vi "Change Camera.vi"() -> ()   [LabVIEW 2015]
uses:
  <vilib>/Rock Robotics/SystemInterfaces/NetworkCommunication/NetComm_UsageReport_ResourceType.ctl
panel:
  in  "error in (no error)":errorcluster
  in  "Switch Camera 2":bool
  in  "Switch Camera":bool
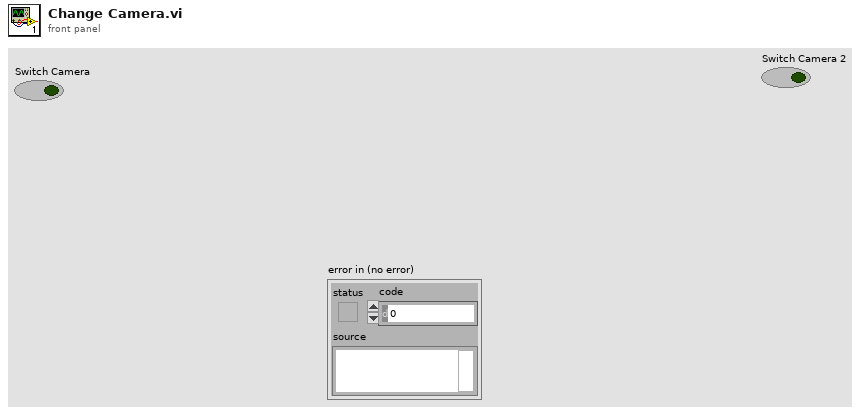
[diagram p1: front panel]
types:
  T1 = cluster{"fps":i32, "compression":i32, "compression 2":i32}
  T2 = typedef "NetComm_UsageReport_ResourceType.ctl" = enum8{"Controller", "Module", "Language", "CANPlugin", "Accelerometer", "ADXL345", "AnalogChannel", "AnalogTrigger", "AnalogTriggerOutput", "CANJaguar", "Compressor", "Counter", "Dashboard", "DigitalInput", "DigitalOutput", "DriverStationCIO", "DriverStationEIO", "DriverStationLCD", "Encoder", "GearTooth", "Gyro", "I2C", "Framework", "Jaguar", "Joystick", "Kinect", "KinectStick", "PIDController", "Preferences", "PWM", "Relay", "RobotDrive", "SerialPort", "Servo", "Solenoid", "SPI", "Task", "Ultrasonic", "Victor", "Button", "Command", "AxisCamera", "PCVideoServer", "SmartDashboard", "Talon", "HiTechnicColorSensor", "HiTechnicAccel", "HiTechnicCompass", "SRF08", "AnalogOutput", "Victor SP", "Talon SRX", "CAN Talon SRX", "ADXL362 Accel", "ADXRS450 Gyro", "Rev SPARK", "Mindsensors SD540", "Digital Filter"}
  T3 = enum16{"Update Mode", "Get Image", "Get Image Data"}
  T4 = typedef "WPI_CameraDevRef.ctl" = cluster{"Camera Address":string, "CameraStatus":errorcluster}
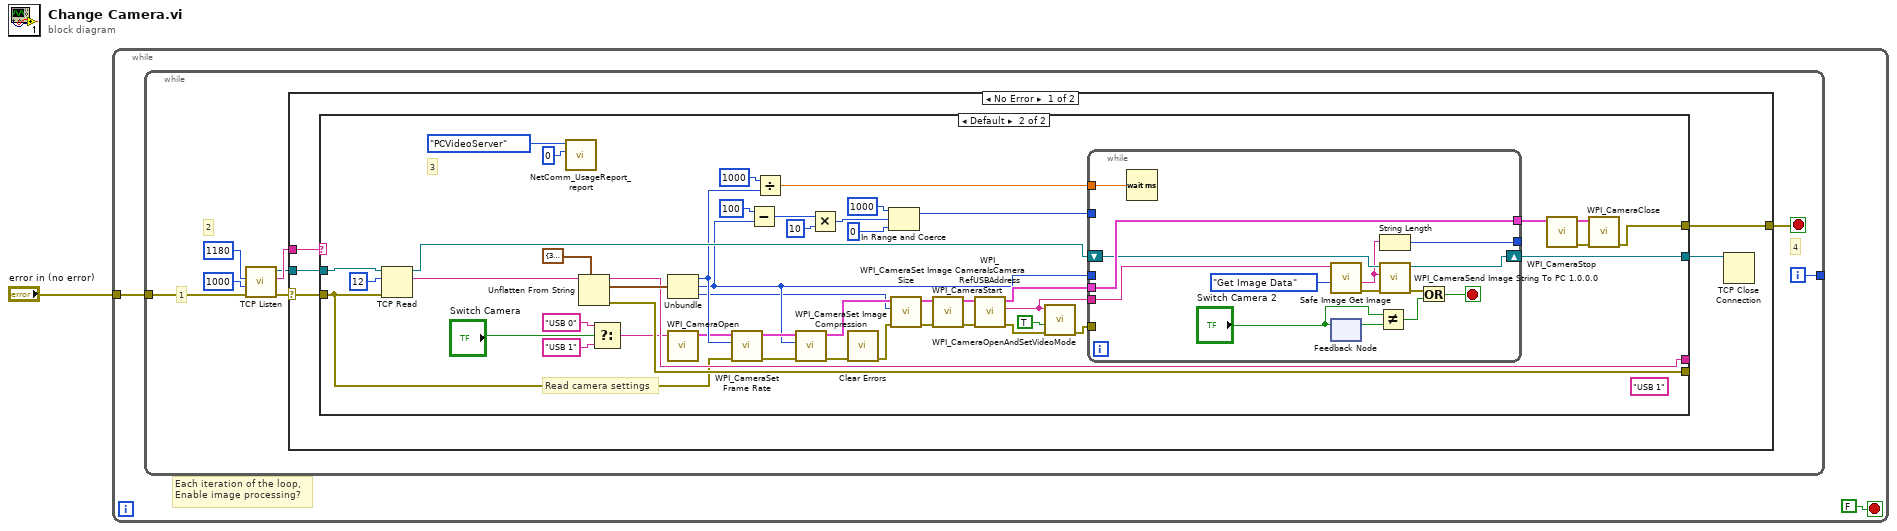
[diagram p0: block diagram]
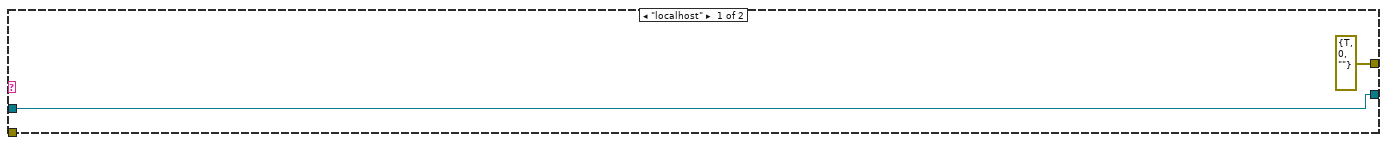
[diagram p2: hidden frame]
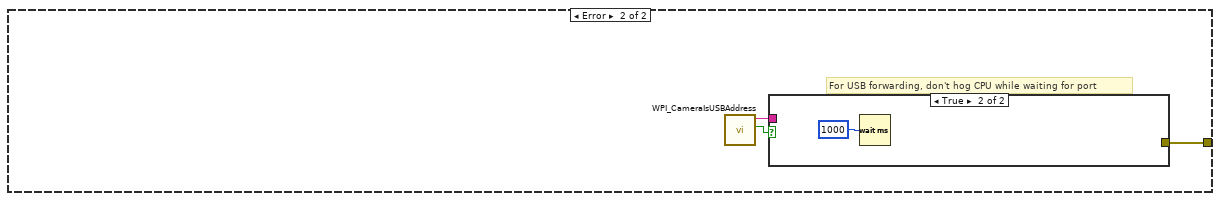
[diagram p3: hidden frame]
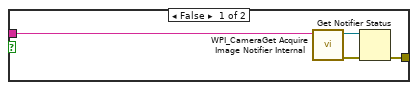
[diagram p4: hidden frame]
diagram:
  n1 = while {
    tunnel: "error in (no error)" -> [w2]
    stop <- FALSE stop-if-true
    # "Each iteration of the loop,\nEnable image processing?"
    n2 = while {
      tunnel: w2 -> [w10]
      tunnel: [w4] -> _
      i -> [w4]
      stop <- w8 stop-if-true
      # "4"
      # "1"
      # "2"
      n3 = call <vilib>:"TCP Listen.vi"("error in (no error)"=w10, "timeout ms (wait forever: -1)"=u16 1000 ("port"), "port"=u16 1180) -> ("error out"=w6:errorcluster, "remote address"=w11:string, "connection ID"=w9:refnum<k5>)  [unwired: 1 in, 5 out]
      n4 = case shown="No Error" w6 {
        selector: w6 -> [w12 _]
        tunnel: w11 -> [w16 _]
        tunnel: w9 -> [w15 _]
        tunnel: [w14 w82] -> w8
        frame No Error {
          n5 = case shown="Default" w16 {
            tunnel: w12 -> [_ w32]
            tunnel: w15 -> [w17 w56]
            tunnel: [errorcluster {"status"=TRUE, "code"=0, "source"=""} ("error out 2") w20] -> w14
            tunnel: [w17 w65] -> w13
            tunnel: [_ w34] -> _
            tunnel: [_ w33] -> _
            frame "localhost" {
            }
            frame Default {
              (unwired) "USB 1" ("format string")
              # "Read camera settings"
              # "3"
              n6 = TCP Read(connection ID=w56, bytes to read=12, error in (no error)=w32) -> (connection ID out=w55:refnum<k5>, data out=w53:string)  [unwired: 2 in, 1 out]
              n7 = call <vilib>:"NetComm_UsageReport_report.vi"("Instance Number"=u8 0, "Resource Type"=NetComm_UsageReport_ResourceType."PCVideoServer") -> ()  [unwired: 10 in]
              n8 = Unflatten From String(type=T1 {"fps"=30, "compression"=32, "compression 2"=32} ("Camera Settings"), binary string=w53) -> (rest of the binary string=w33:string, value=w47:T1, error out=w34:errorcluster)  [unwired: 3 in]
              n9 = Select(t="USB 0" ("format string"), s="Switch Camera", f="USB 1" ("format string")) -> (s? t:f=w22:string)
              n10 = Unbundle(w47) -> ("fps"=w31:i32, "compression"=w30:i32, "compression 2"=w29:i32)
              n11 = call <vilib>:"WPI_CameraOpen.vi"("Camera Address"=w22) -> ("CameraDevRef"=w21:T4)  [unwired: 1 in, 9 out]
              n12 = call <vilib>:"WPI_CameraSet Frame Rate.vi"("error in (no error)"=w32, "Frame Rate (fps)"=w31, "CameraDevRef"=w21) -> ("error out"=w49:errorcluster, "CameraDevRef Out"=w52:T4)  [unwired: 7 in]
              n13 = Subtract(x=100, y=w30) -> (x-y=w40:i32)
              n14 = Divide(x=u16 1000 ("port"), y=w31) -> (x/y=w45:dbl)
              n15 = call <vilib>:"WPI_CameraSet Image Compression.vi"("error in (no error)"=w49, "Compression"=w30, "CameraDevRef"=w52) -> ("error out"=w36:errorcluster, "CameraDevRef Out"=w51:T4)  [unwired: 7 in]
              n16 = Multiply(x=w40, y=10) -> (x*y=w42:i32)
              n17 = call <vilib>:"Clear Errors.vi"("error in (no error)"=w36) -> ("error out"=w35:errorcluster)  [unwired: 5 in, 1 out]
              n18 = In Range and Coerce(upper limit=1000, x=w42, lower limit=0) -> (coerced(x)=w38:i32)  [unwired: 1 out]
              n19 = call <vilib>:"WPI_CameraSet Image Size.vi"("error in (no error)"=w35, "Image Size"=w29, "CameraDevRef"=w51) -> ("error out"=w48:errorcluster, "CameraDevRef Out"=w50:T4)  [unwired: 7 in]
              n20 = call <vilib>:"WPI_CameraStart.vi"("error in (no error)"=w48, "CameraDevRef"=w50) -> ("error out"=w60:errorcluster, "CameraDevRef"=w58:T4)  [unwired: 8 out]
              n21 = call <vilib>:"WPI_CameraIsCameraRefUSBAddress.vi"("error in (no error)"=w60, "CameraDevRef"=w58) -> ("error out"=w59:errorcluster, "Camera Address Out"=w61:string, "CameraDevRef out"=w57:T4)  [unwired: 6 in, 1 out]
              n22 = call <vilib>:"WPI_CameraOpenAndSetVideoMode.vi"("error in (no error)"=w59, "USB JPEG"=TRUE, "Camera Address Out"=w61) -> ("error out"=w28:errorcluster)  [unwired: 8 in]
              n23 = while {
                tunnel: w61 -> [w67]
                shift-right: [w79] -> w65
                shift-left: w55 -> [w76]
                tunnel: [w78] -> w64
                tunnel: w57 -> [w78]
                tunnel: w38 -> [_]
                tunnel: w45 -> [w77]
                tunnel: [w75] -> _
                tunnel: w30 -> [_]
                tunnel: w28 -> [_]
                stop <- w68 stop-if-true
                n24 = Wait (ms)(milliseconds to wait=w77) -> ()  [unwired: 1 out]
                n25 = call <vilib>:"Safe Image Get Image.vi"("Operation"=T3."Get Image Data", "Session In"=w67) -> ("error out"=w72:errorcluster, "Image Data String"=w73:string)  [unwired: 6 in, 2 out]
                n26 = feedback-in #1("Switch Camera 2") -> ()
                n27 = feedback #1() -> (w71:bool)  [unwired: 1 in]
                n28 = Not Equal?(x="Switch Camera 2", y=w71) -> (x != y?=w70:bool)
                n29 = String Length(string=w73) -> (length=w75:i32)
                n30 = call <vilib>:"WPI_CameraSend Image String To PC 1.0.0.0.vi"("error in (no error)"=w72, "String"=w73, "TCP Connection ID"=w76) -> ("error out"=w69:errorcluster, "TCP Connection ID out"=w79:refnum<k5>)  [unwired: 7 out]
                n31 = Or(x=w69, y=w70) -> (x .or. y?=w68:bool)
              }
              n32 = call <vilib>:"WPI_CameraStop.vi"("CameraDevRef"=w64) -> ("error out"=w25:errorcluster, "CameraDevRef"=w26:T4)  [unwired: 1 in, 8 out]
              n33 = call <vilib>:"WPI_CameraClose.vi"("error in (no error)"=w25, "CameraDevRef"=w26) -> ("error out"=w20:errorcluster)  [unwired: 9 in]
            }
          }
          n34 = TCP Close Connection(connection ID=w13) -> ()  [unwired: 1 in, 3 out]
        }
        frame Error {
          # "For USB forwarding, don't hog CPU while waiting for port"
          n35 = call <vilib>:"WPI_CameraIsUSBAddress.vi"() -> ("USB?"=w80:bool, "Camera Address Out"=w81:string)  [unwired: 9 in, 1 out]
          n36 = case shown="True" w80 {
            tunnel: [w86 _] -> w82
            tunnel: w81 -> [w83 _]
            frame False {
              n37 = call <vilib>:"WPI_CameraGet Acquire Image Notifier Internal.vi"("Camera Address"=w83) -> ("error out"=w84:errorcluster, "Acquire Image Notifier"=w85:refnum<notifier>)  [unwired: 1 in, 8 out]
              n38 = Get Notifier Status(notifier=w85, error in (no error)=w84) -> (error out=w86:errorcluster)  [unwired: 4 out]
            }
            frame True {
              n39 = Wait (ms)(milliseconds to wait=u32 1000) -> ()  [unwired: 1 out]
            }
          }
        }
      }
    }
  }
